vi "check targets.vi"(8 "error in":errorcluster, 11 "Targets In":T1) -> (0 "error in 2":errorcluster)   [LabVIEW 2016]
panel:
  out "Targets Out":T1
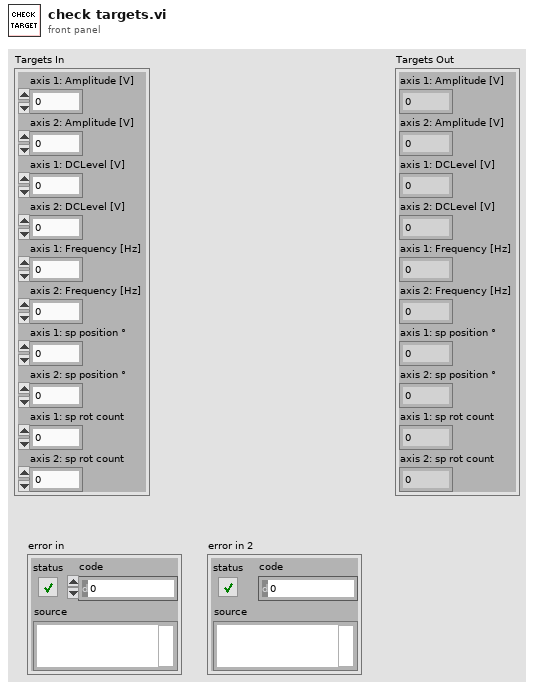
[diagram p1: front panel]
types:
  T1 = cluster{"axis 1: Amplitude [V]":dbl, "axis 2: Amplitude [V]":dbl, "axis 1: DCLevel [V]":dbl, "axis 2: DCLevel [V]":dbl, "axis 1: Frequency [Hz]":dbl, "axis 2: Frequency [Hz]":dbl, "axis 1: sp position °":dbl, "axis 2: sp position °":dbl, "axis 1: sp rot count":dbl, "axis 2: sp rot count":dbl}
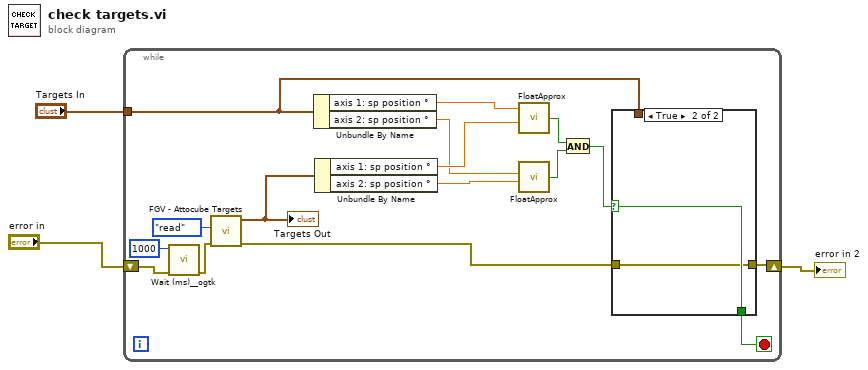
[diagram p0: block diagram]
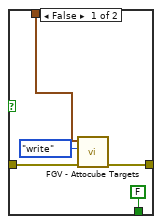
[diagram p2: hidden frame]
diagram:
  n1 = while {
    tunnel: "Targets In" -> [w7]
    shift-right: [w8] -> w1
    shift-left: "error in" -> [w6]
    stop <- w10 stop-if-true
    n2 = call <userlib>:"Wait (ms)__ogtk.vi"("error in (no error)"=w6, "milliseconds to wait"=u32 1000) -> ("error out"=w5:errorcluster)  [unwired: 8 in, 1 out]
    n3 = call "FGV - Attocube Targets.vi"("error in"=w5, "Function"=enum16{"write", "read"}."read") -> ("error out"=w9:errorcluster, "Targets Out"=w18:T1)  [unwired: 4 in]
    "Targets Out" <- w18
    n4 = Unbundle By Name(w7) -> ("axis 1: sp position °"=w17:dbl, "axis 2: sp position °"=w15:dbl)
    n5 = Unbundle By Name(w18) -> ("axis 1: sp position °"=w16:dbl, "axis 2: sp position °"=w14:dbl)
    n6 = call <userlib>:"FloatApprox.vi"("y"=w16, "x"=w17) -> ("x ~ y?"=w13:bool)  [unwired: 2 in]
    n7 = call <userlib>:"FloatApprox.vi"("y"=w14, "x"=w15) -> ("x ~ y?"=w12:bool)  [unwired: 2 in]
    n8 = And(x=w13, y=w12) -> (x .and. y?=w11:bool)
    n9 = case shown="True" w11 {
      selector: w11 -> [_ w26]
      tunnel: [FALSE w26] -> w10
      tunnel: w9 -> [w24 w25]
      tunnel: [w23 w25] -> w8
      tunnel: w7 -> [w20 _]
      frame False {
        n10 = call "FGV - Attocube Targets.vi"("error in"=w24, "Function"=enum16{"write", "read"}."write", "Targets In"=w20) -> ("error out"=w23:errorcluster)  [unwired: 3 in, 1 out]
      }
      frame True {
      }
    }
  }
  "error in 2" <- w1
